vi "模式删除面板.vi"(10 "pannel-id":dbl, 11 "模式 input":T1 {"sce-pannel-list"."pannel"."ID" format="%02x"}) -> (3 "模式 output":T1 {"sce-pannel-list"."pannel"."ID" format="%02x"})   [LabVIEW 2019]
panel:
  in  "模式选择":string(combo)
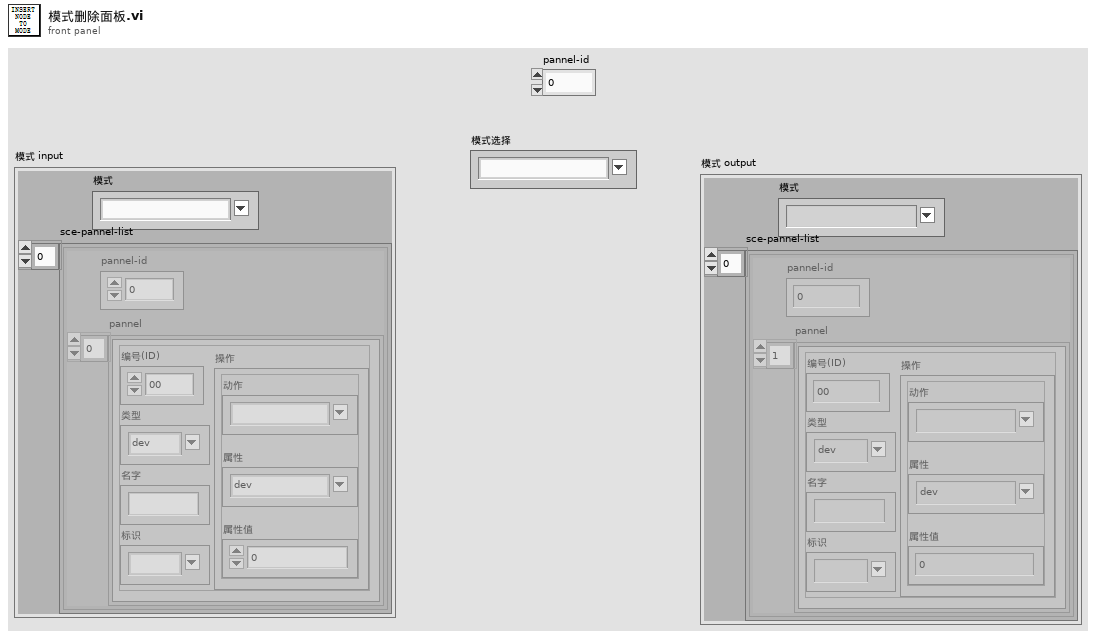
[diagram p1: front panel]
types:
  T1 = cluster{"模式":string, "sce-pannel-list":cluster{"pannel":cluster{"ID":u8, "type":string, "flag":string, "name":string, "Act":cluster{"Attribute":string, "Action":string, "Value":dbl}}[], "pannel-id":dbl}[]}
  T2 = cluster{"pannel":cluster{"ID":u8, "type":string, "flag":string, "name":string, "Act":cluster{"Attribute":string, "Action":string, "Value":dbl}}[], "pannel-id":dbl}[]
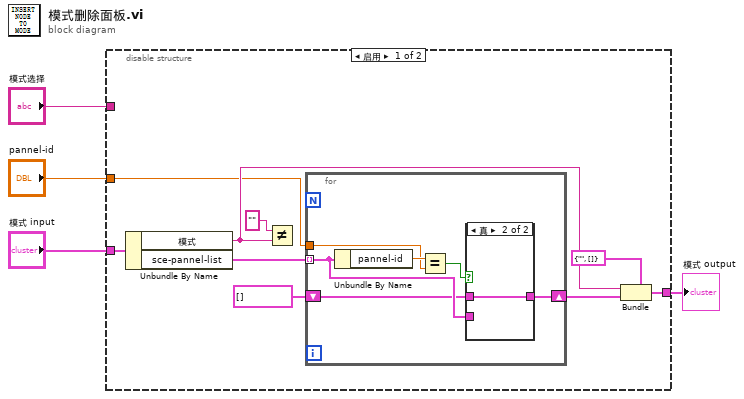
[diagram p0: block diagram]
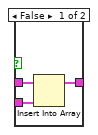
[diagram p2: hidden frame]
diagram:
  n1 = disable-structure shown="启用" {
    disable-tunnel: "模式 input" -> [w10 _]
    disable-tunnel: "模式选择" -> [_ _]
    disable-tunnel: [w9 _] -> w2
    disable-tunnel: "pannel-id" -> [w6 _]
    frame Enabled {
      n2 = Unbundle By Name(w10) -> ("模式"=w12:string, "sce-pannel-list"=w13:T2)
      n3 = Not Equal?(x="", y=w12) -> ()  [unwired: 1 out]
      n4 = for {
        tunnel: w13 -> [w17] mode=indexing
        shift-right: [w16] -> w5
        shift-left: T2 [] -> [w15]
        tunnel: w6 -> [w14]
        n5 = Unbundle By Name(w17) -> ("pannel-id"=w19:dbl)
        n6 = Equal?(x=w19, y=w14) -> (x = y?=w18:bool)
        n7 = case shown="真" w18 {
          tunnel: w17 -> [w22 _]
          tunnel: [w21 w23] -> w16
          tunnel: w15 -> [w20 w23]
          frame False {
            n8 = Insert Into Array(array=w20, new element=w22) -> (w21:T2)  [unwired: 1 in]
          }
          frame True {
          }
        }
      }
      n9 = Bundle(cluster=T1 {"模式"="", "sce-pannel-list"=[]} ("模式 input"), "模式"=w12, "sce-pannel-list"=w5) -> (w9:T1)
    }
    frame Disabled {
    }
  }
  "模式 output" <- w2
